vi "base_del_triangulo.vi"() -> ()   [LabVIEW 2020]
panel:
  out "Numeric 3":dbl
  in  "Numeric 2":dbl
  in  "Numeric":dbl
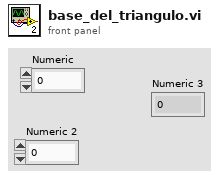
[diagram p1: front panel]
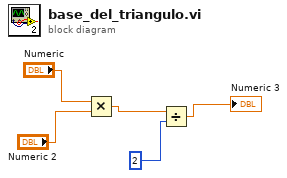
[diagram p0: block diagram]
diagram:
  n1 = Multiply(x="Numeric", y="Numeric 2") -> (x*y=w3:dbl)
  n2 = Divide(x=w3, y=2) -> (x/y=→"Numeric 3":dbl)
